vi "Fassade 1.vi"(0 "Data In":T4 caption="Daten (Eingang)", 2 "Display State In":T2 caption="Anzeigezustand (Eingang)", 3 "Container State":T3 caption="Container-Status") -> (6 "Data Out":T4 caption="Daten (Ausgang)", 7 "Display State Out":T2 caption="Anzeigezustand (Ausgang)", 8 "Action":T1 caption="Aktion")   [LabVIEW 2010, in "util.lvlib" / "XControl 1.xctl"]
uses:
  XControl 1.xctl
  Daten 1.ctl
  <vilib>/_xctls/Container State.ctl
  Zustand 1.ctl
  <vilib>/_xctls/Action.ctl
  <vilib>/_xctls/XControlSupport.lvlib
panel:
  # "1. Legen Sie die Elemente für das Erscheinungsbild \ndes XControls hier ab.\n\n2. Ändern Sie die Größe des Fensters bezüglich der Elemente\n\n3. Wenn das XControl eine feste Größe haben soll,   \n legen Sie dies unter VI-Einstellungen->Fenstererscheinungsbild fest.\n\n4. Wenn die Elemente ihre Größe ändern sollen, wenn das XControl seine Größe verändert, setzen Sie die Option  \"Alle Objekte auf Frontpanel bei Größenänderung des Fensters neu skalieren\" unter Datei->VI-Einstellungen->Fenstergröße.\n\n5. Wechseln Sie auf das Blockdiagramm und bearbeiten Sie die zu behandelnden Ereignisse."
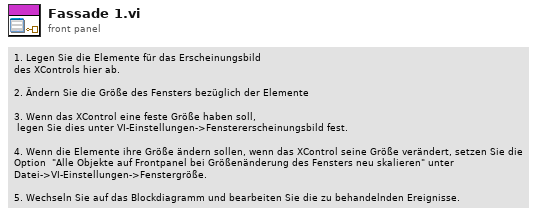
[diagram p1: front panel]
types:
  T1 = typedef "XControlSupport.lvlib/Action.ctl" = cluster{"Data Changed?":bool, "State Changed?":bool, "Action Name":string}
  T2 = typedef "util.lvlib/XControl 1.xctl/Zustand 1.ctl" = cluster{"Numeric":dbl}
  T3 = typedef "XControlSupport.lvlib/Container State.ctl" = cluster{"Indicator?":bool, "Run Mode?":bool, " Refnum":refnum<vi>}
  T4 = typedef "util.lvlib/XControl 1.xctl/Daten 1.ctl" = dbl
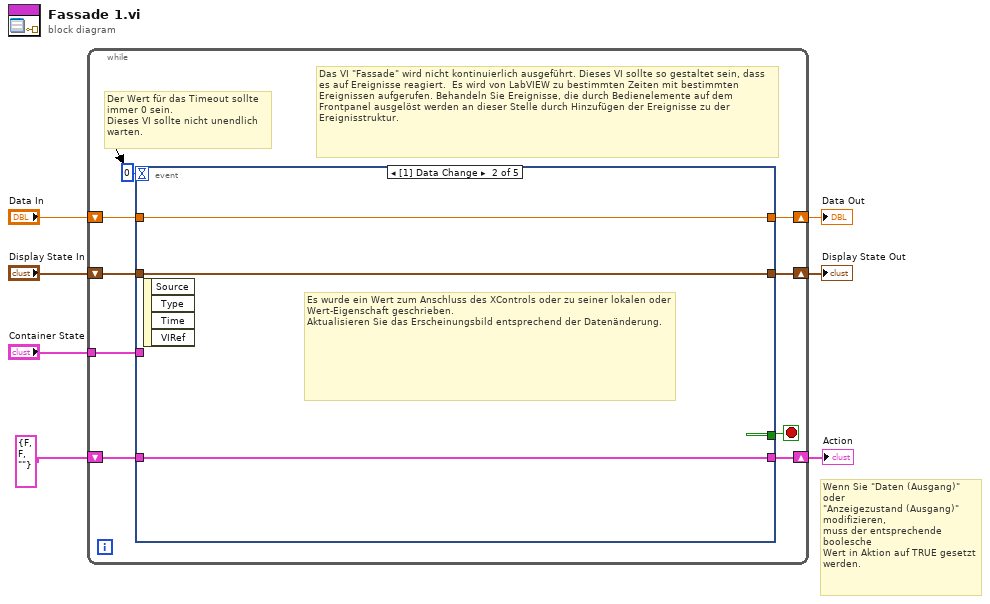
[diagram p0: block diagram]
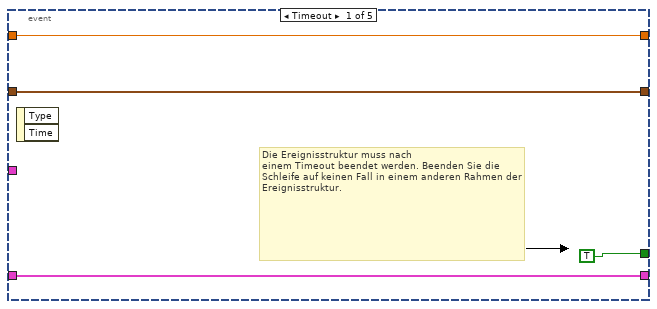
[diagram p2: hidden frame]
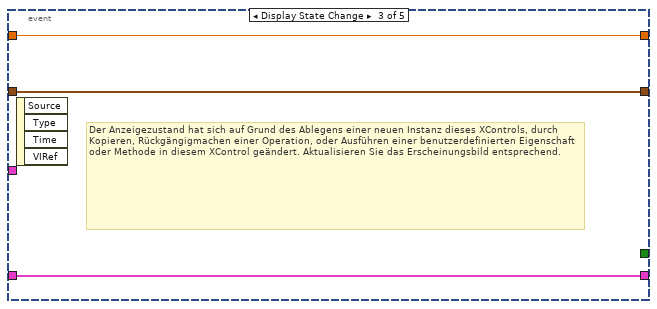
[diagram p3: hidden frame]
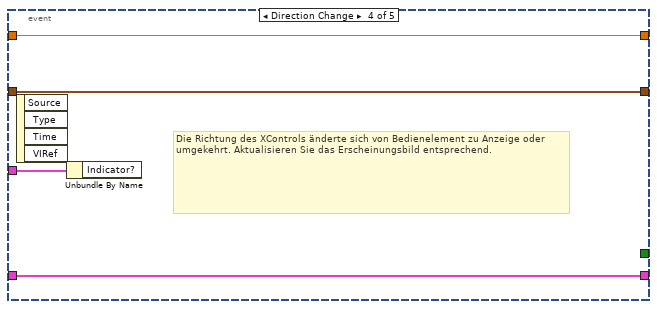
[diagram p4: hidden frame]
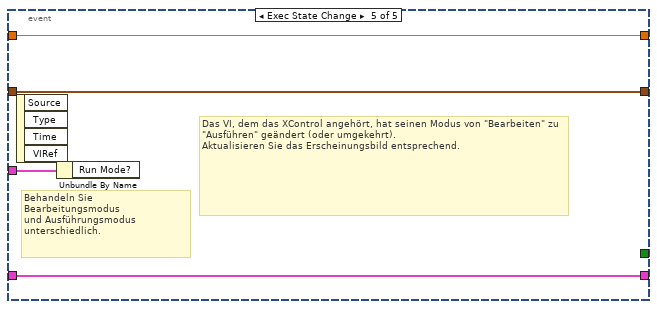
[diagram p5: hidden frame]
diagram:
  # "Wenn Sie \"Daten (Ausgang)\" oder\n\"Anzeigezustand (Ausgang)\" modifizieren,\nmuss der entsprechende boolesche\nWert in Aktion auf TRUE gesetzt werden."
  n1 = while {
    shift-right: [w15] -> w4
    shift-left: "Display State In" -> [w16]
    tunnel: "Container State" -> [w12]
    shift-right: [w10] -> w7
    shift-left: "Data In" -> [w11]
    shift-right: [w8] -> w2
    shift-left: T1 {"Data Changed?"=FALSE, "State Changed?"=FALSE, "Action Name"=""} ("Action") -> [w9]
    stop <- w14 stop-if-true
    # "Das VI \"Fassade\" wird nicht kontinuierlich ausgeführt. Dieses VI sollte so gestaltet sein, dass es auf Ereignisse reagiert.  Es wird von LabVIEW zu bestimmten Zeiten mit bestimmten Ereignissen aufgerufen. Behandeln Sie Ereignisse, die durch Bedienelemente auf dem Frontpanel ausgelöst werden an dieser Stelle durch Hinzufügen der Ereignisse zu der Ereignisstruktur."
    # "Der Wert für das Timeout sollte immer 0 sein. \nDieses VI sollte nicht unendlich warten."
    n2 = event shown="[1] Data Change" {
      selector: _ -> [_ _ _ _ _]
      dyn-events: _ -> [_ _ _ _ _]
      timeout: 0 -> [_ _ _ _ _]
      tunnel: w16 -> [w18 w22 w26 w29 w33]
      tunnel: [w18 w22 w26 w29 w33] -> w15
      tunnel: [TRUE _ _ _ _] -> w14
      tunnel: w12 -> [_ _ _ w30 w34]
      tunnel: w11 -> [w17 w23 w25 w28 w32]
      tunnel: [w17 w23 w25 w28 w32] -> w10
      tunnel: [w19 w21 w24 w27 w31] -> w8
      tunnel: w9 -> [w19 w21 w24 w27 w31]
      event Timeout {
        # "Die Ereignisstruktur muss nach\neinem Timeout beendet werden. Beenden Sie die Schleife auf keinen Fall in einem anderen Rahmen der Ereignisstruktur."
        n3 = event-data() -> ()  [unwired: 1 in, 2 out]
      }
      event Data Change {
        # "Es wurde ein Wert zum Anschluss des XControls oder zu seiner lokalen oder Wert-Eigenschaft geschrieben.\nAktualisieren Sie das Erscheinungsbild entsprechend der Datenänderung."
        n4 = event-data() -> ()  [unwired: 1 in, 4 out]
      }
      event Display State Change {
        # "Der Anzeigezustand hat sich auf Grund des Ablegens einer neuen Instanz dieses XControls, durch Kopieren, Rückgängigmachen einer Operation, oder Ausführen einer benutzerdefinierten Eigenschaft oder Methode in diesem XControl geändert. Aktualisieren Sie das Erscheinungsbild entsprechend."
        n5 = event-data() -> ()  [unwired: 1 in, 4 out]
      }
      event Direction Change {
        # "Die Richtung des XControls änderte sich von Bedienelement zu Anzeige oder umgekehrt. Aktualisieren Sie das Erscheinungsbild entsprechend."
        n6 = event-data() -> ()  [unwired: 1 in, 4 out]
        n7 = Unbundle By Name(w30) -> ()  [unwired: 1 out]
      }
      event Exec State Change {
        # "Das VI, dem das XControl angehört, hat seinen Modus von \"Bearbeiten\" zu \"Ausführen\" geändert (oder umgekehrt).\nAktualisieren Sie das Erscheinungsbild entsprechend."
        # "Behandeln Sie Bearbeitungsmodus\nund Ausführungsmodus unterschiedlich."
        n8 = event-data() -> ()  [unwired: 1 in, 4 out]
        n9 = Unbundle By Name(w34) -> ()  [unwired: 1 out]
      }
    }
  }
  "Display State Out" <- w4
  "Data Out" <- w7
  "Action" <- w2
